vi "Com_SECS Equipment _Data Message_U2.vi"(7 "Parent Index":i32=-1, 8 "error in":errorcluster, 10 "Data":u16[](array[numeric]), 11 "Message Data In":T1[](array[typedef])) -> (0 "error out":errorcluster, 3 "Message Data Out":T1[](array[typedef]))   [LabVIEW 2016]
uses:
  Data Def/Com_SECS Equipment _Message Data.ctl
  Data Def/Com_SECS Equipment _Data Item Format.ctl
  Data Def/Com_SECS Equipment _Format Code.ctl
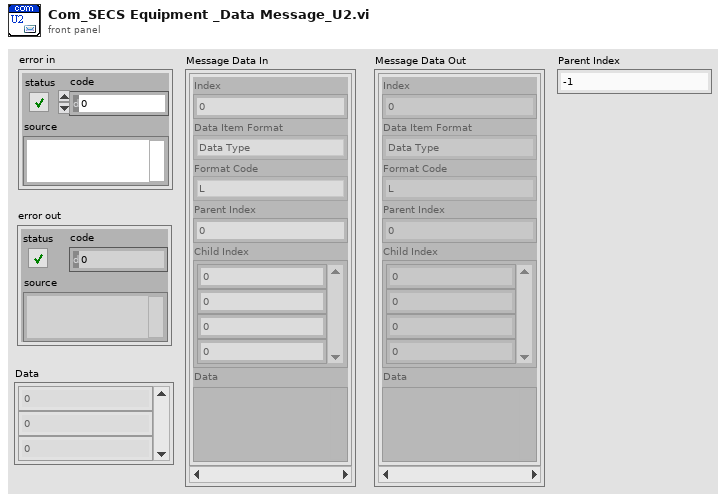
[diagram p1: front panel]
types:
  T1 = typedef "Com_SECS Equipment _Message Data.ctl" = cluster{"Index":i32, "Data Item Format":T2, "Format Code":T3, "Parent Index":i32, "Child Index":i32[], "Data":variant}
  T2 = typedef "Com_SECS Equipment _Data Item Format.ctl" = enum16{"Data Type", "Value"}
  T3 = typedef "Com_SECS Equipment _Format Code.ctl" = enum16{"L", "A", "B", "Boolean", "J", "I1", "I2", "I4", "I8", "U1", "U2", "U4", "U8", "F4", "F8", "Char"}
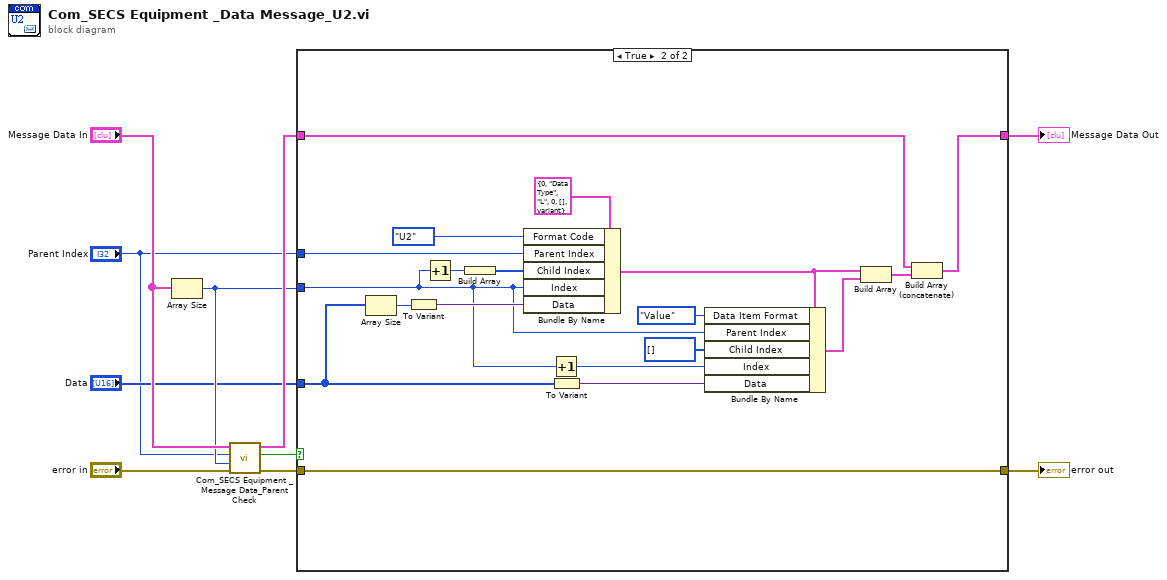
[diagram p0: block diagram]
diagram:
  n1 = Array Size(array="Message Data In") -> (size(s)=w5:i32)
  n2 = call "Com_SECS Equipment _Message Data_Parent Check.vi"("error in"="error in", "Message Index"=w5, "Parent Index"="Parent Index", "Message Data In"="Message Data In") -> ("error out"=w8:errorcluster, "OK?"=w9:bool, "Message Data Out"=w6:T1[])  [unwired: 5 in]
  n3 = case shown="True" w9 {
    tunnel: w8 -> [w11 w15]
    tunnel: w6 -> [w12 w17]
    tunnel: [w12 w16] -> w4
    tunnel: "Parent Index" -> [_ w24]
    tunnel: w5 -> [_ w14]
    tunnel: "Data" -> [_ w13]
    tunnel: [w11 w15] -> w3
    frame False {
    }
    frame True {
      n4 = Array Size(array=w13) -> (size(s)=w27:i32)
      n5 = To Variant(anything=w27) -> (Variant=w26:variant)
      n6 = Increment(x=w14) -> (x+1=w29:i32)
      n7 = Build Array(w29) -> (w28:i32[])
      n8 = Bundle By Name(cluster=T1 {"Index"=0, "Data Item Format"=enum."Data Type", "Format Code"=enum."L", "Parent Index"=0, "Child Index"=[], "Data"=variant} ("Message Data"), "Format Code"=Com_SECS_Equipment__Format_Code."U2", "Parent Index"=w24, "Child Index"=w28, "Index"=w14, "Data"=w26) -> (w20:T1)
      n9 = Increment(x=w14) -> (x+1=w22:i32)
      n10 = To Variant(anything=w13) -> (Variant=w21:variant)
      n11 = Bundle By Name(cluster=w20, "Data Item Format"=Com_SECS_Equipment__Data_Item_Format."Value", "Parent Index"=w14, "Child Index"=i32[] [], "Index"=w22, "Data"=w21) -> (w19:T1)
      n12 = Build Array(w20, w19) -> (w18:T1[])
      n13 = Build Array (concatenate)(w17, w18) -> (w16:T1[])
    }
  }
  "error out" <- w3
  "Message Data Out" <- w4
